vi "Update Tag Double.vi"(8 "error in (no error)":errorcluster, 9 "Value":dbl, 10 "Tag Path":string, 11 "Logger in.lvclass":refnum<class "Logger.lvclass">) -> (0 "error out":errorcluster, 3 "Logger out.lvclass":refnum<class "Logger.lvclass">)   [LabVIEW 2017, in "Logger.lvclass"]
uses:
  Logger.lvclass
  Logger.lvclass/Logger.ctl
  <vilib>/Skyline/Tag/Wrapper/Wrapper_class/Generate Tag Cluster (DBL).vi
  <vilib>/Skyline/Tag/Wrapper/Wrapper_class/NI Skyline Tag.lvclass
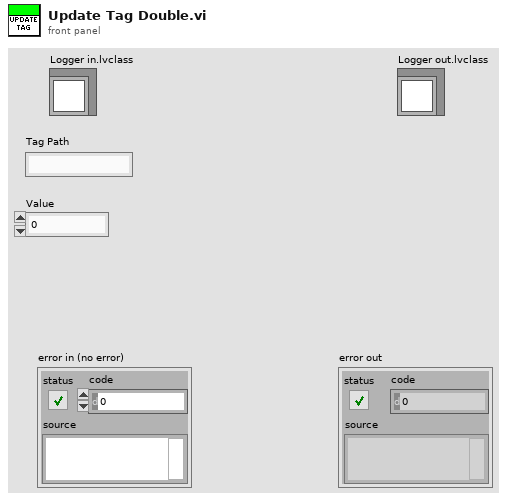
[diagram p1: front panel]
types:
  T1 = cluster{"Tag Units":string, "Tag Path":string, "Waveform":waveform(dbl), "Log":bool, "Tag Reference":refnum<class "NI Skyline Tag.lvclass">}[]
  T2 = typedef "NI Skyline Tag.lvlib/Tag Cluster Wrapper.ctl" = cluster{"Configuration":refnum<class "NI Skyline Configuration.lvclass">, "Tag Cluster":T3}
  T3 = typedef "NI Skyline Tag.lvlib/Tag Cluster.ctl" = cluster{"Path":string, "Data Type":T4, "Value":variant, "Time Stamp":timestamp}
  T4 = typedef "NI Skyline Tag.lvlib/DataType.ctl" = enum32{"Double", "Integer", "String"}
  T5 = cluster{"Tag Units":string, "Tag Path":string, "Waveform":waveform(dbl), "Log":bool, "Tag Reference":refnum<class "NI Skyline Tag.lvclass">}
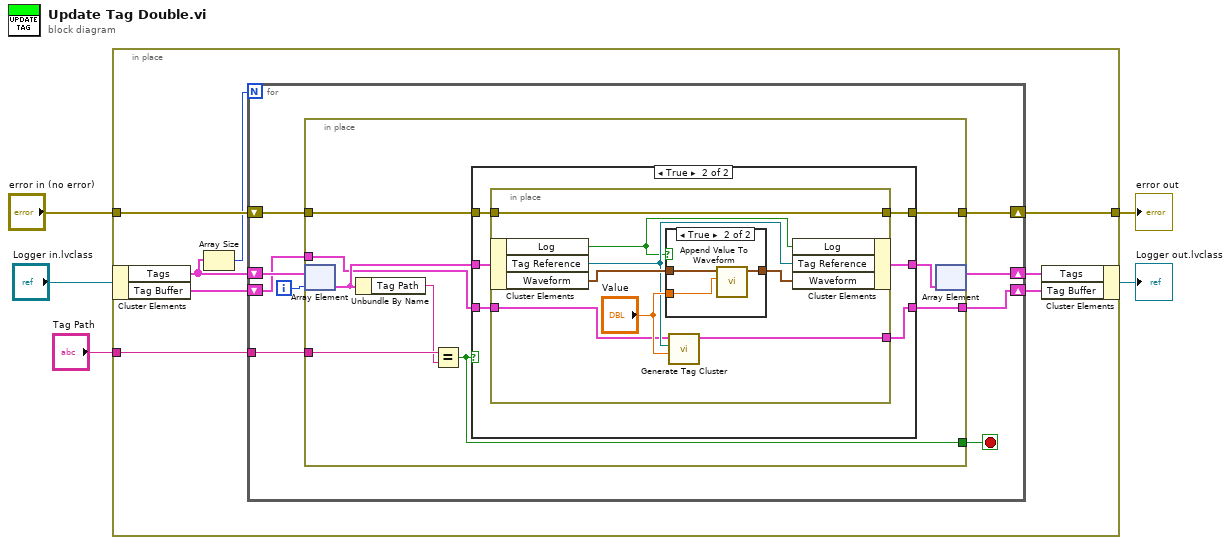
[diagram p0: block diagram]
diagram:
  n1 = in-place {
    in-place-border: "Tag Path" -> [w13]
    in-place-border: "error in (no error)" -> [w11]
    in-place-border: [w10] -> w1
    n2 = in-place-cluster #1("Logger in.lvclass") -> ("Tags"=w8:T1, "Tag Buffer"=w7:T2[])
    n3 = Array Size(array=w8) -> (size(s)=w9:i32)
    n4 = for {
      N: w9 -> [_]
      tunnel: w13 -> [w22]
      shift-right: [w19] -> w12
      shift-left: w8 -> [w21]
      shift-right: [w17] -> w10
      shift-left: w11 -> [w18]
      shift-right: [w14] -> w6
      shift-left: w7 -> [w15]
      i -> [w20]
      stop <- w16 stop-if-true
      n5 = in-place {
        in-place-border: w22 -> [w27]
        in-place-border: [w25] -> w16
        in-place-border: w18 -> [w29]
        in-place-border: [w28] -> w17
        in-place-border: w15 -> [w24]
        in-place-border: [w23] -> w14
        n6 = in-place-array #2(w21, w20) -> (w30:T5)
        n7 = Unbundle By Name(w30) -> ("Tag Path"=w26:string)
        n8 = Equal?(x=w27, y=w26) -> (x = y?=w25:bool)
        n9 = case shown="True" w25 {
          tunnel: w30 -> [w34 w40]
          tunnel: [w34 w39] -> w31
          tunnel: w29 -> [w33 w38]
          tunnel: [w33 w35] -> w28
          tunnel: w24 -> [w32 w37]
          tunnel: [w32 w36] -> w23
          frame False {
          }
          frame True {
            n10 = in-place {
              in-place-border: w38 -> [w44]
              in-place-border: w37 -> [w42]
              in-place-border: [w41] -> w36
              in-place-border: [w44] -> w35
              n11 = in-place-cluster #3(w40) -> ("Log"=w43:bool, "Tag Reference"=w45:refnum<class "NI Skyline Tag.lvclass">, "Waveform"=w48:waveform(dbl))
              n12 = case shown="True" w43 {
                tunnel: w48 -> [w49 w52]
                tunnel: [w49 w51] -> w47
                tunnel: "Value" -> [_ w50]
                frame False {
                }
                frame True {
                  n13 = call "Append Value To Waveform.vi"("Numeric"=w50, "waveform in"=w52) -> ("waveform out"=w51:waveform(dbl))  [unwired: 9 in]
                }
              }
              n14 = call-poly <vilib>:"Generate Tag Cluster.vi"("value"="Value", "tag in"=w45, "tag clusters in"=w42) -> ("tag clusters out"=w41:T2[])  [unwired: 6 in, 2 out]
              n15 = in-place-cluster #3("Log"=w43, "Tag Reference"=w45, "Waveform"=w47) -> (w39:T5)
            }
          }
        }
        n16 = in-place-array #2(w31) -> (w19:T1)  [unwired: 1 out]
      }
    }
    n17 = in-place-cluster #1("Tags"=w12, "Tag Buffer"=w6) -> (→"Logger out.lvclass":refnum<class "Logger.lvclass">)
  }
  "error out" <- w1
